vi "yolo-detect-image.vi"() -> ()   [LabVIEW 2017]
uses:
  <vilib>/httpClient/POSTBuffer.vi
  <vilib>/httpClient/LabVIEWHTTPClient.lvlib
panel:
  out "body":string
  out "headers":string
  in  "error in (no error)":errorcluster
  in  "yolo-server \"detect \"endpoint":string="http://localhost:18080/detect"
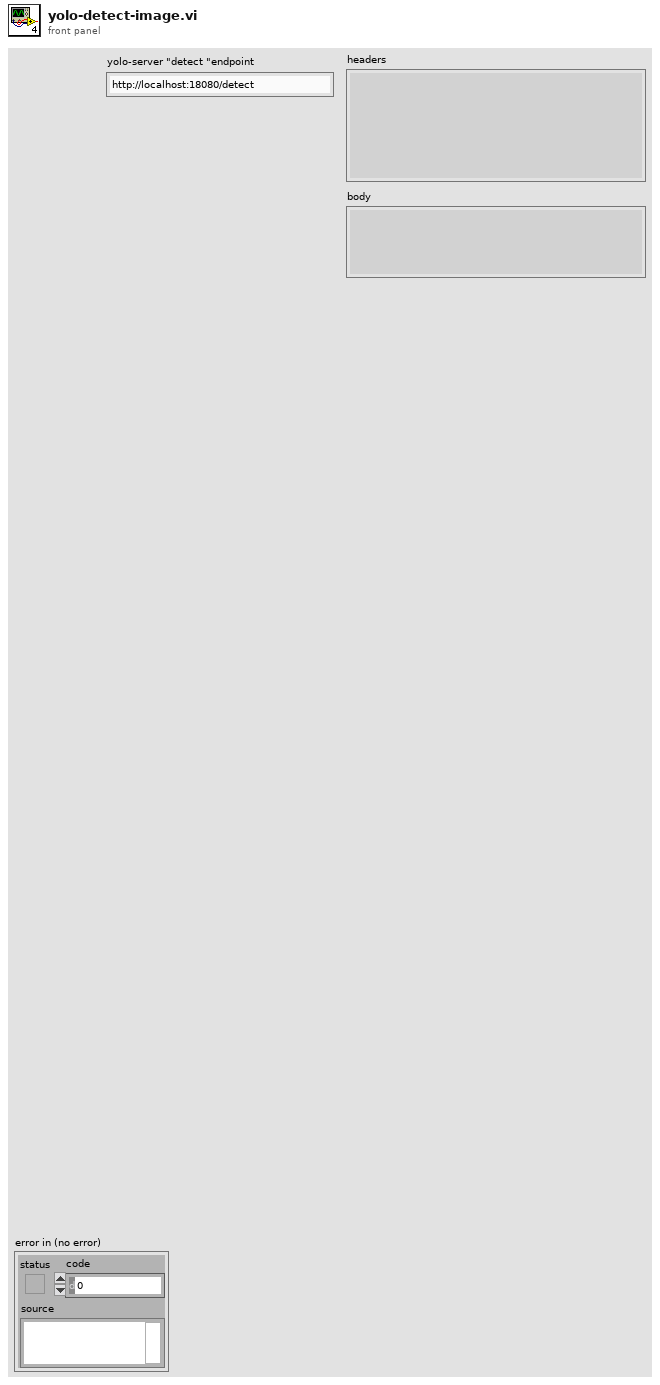
[diagram p1: front panel]
types:
  T1 = typedef "LabVIEWHTTPClient.lvlib/ClientHandle.ctl" = refnum<k1>
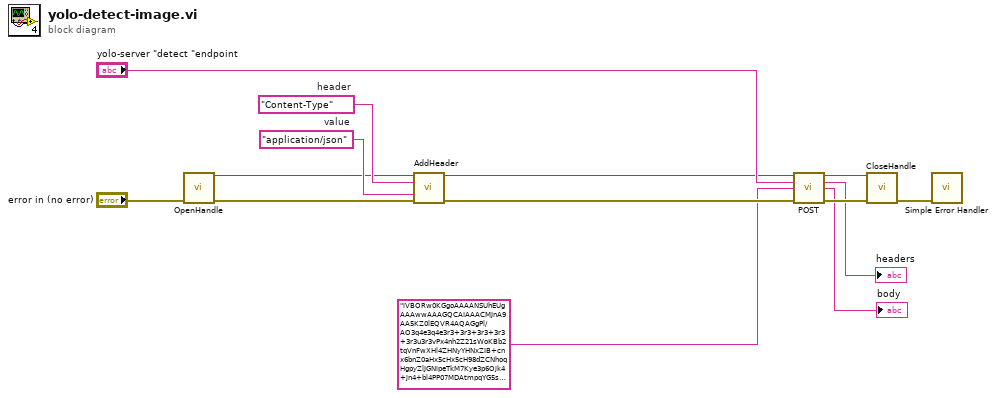
[diagram p0: block diagram]
diagram:
  w14 = "application/json"  # value
  w13 = "Content-Type"  # header
  n1 = call <vilib>:"OpenHandle.vi"("error in (no error)"="error in (no error)") -> ("client handle out"=w7:T1, "error out"=w8:errorcluster)  [unwired: 13 in]
  n2 = call <vilib>:"AddHeader.vi"("client handle"=w7, "header"=w13, "value"=w14, "error in (no error)"=w8) -> ("client handle out"=w4:T1, "error out"=w3:errorcluster)  [unwired: 10 in]
  n3 = call-poly <vilib>:"POST.vi"("client handle"=w4, "url"="yolo-server \"detect \"endpoint", "buffer"="iVBORw0KGgoAAAANSUhEUgAAAwwAAAGQCAIAAACMJnA9AA5KZ0lEQVR4AQAGgPl/AO3q4e3q4e3r3+3r3+3r3+3r3+3r3u3r3vPx4nh2Z21sWoKBb2tqVnFwXHl4ZHNyYHNxZIB+cnx6bnZ0aHx5cHx5cH98dZCNhoqHgpyZlJGNipeTkM7Kye3p6Ojk4+jn4+bl4PP07MDAtmpqYG5sYMLAs+7o3NbQwJ+Wh52VgqqdjKuei7KjjpmKdY5+Z87BrsS+sn16cUJCOikqIh8gGiIlHiMmHxcaERQUDDc1KV5YTJ6VhrWol6WWgbKgirKgiLSeibmkj7ahjq2ciLSjk7msnKeZjId9cauimaqmnXVya2ZnYWBgXmlraIaKiVZVUTAmHDgoGT8vIHNkUcu8p7ChirOli7Oli7SmjLyulL2ul7mqlbytmriomJeHemxeUZCJeYiGd1JTS0BHQEdSTn6JhVtgWSQkGC4mEzMkDUMvFLWhhsCwl4yBa353Z7CtnLGwnrK0n6+woKOnmJuhk5aglZCckoeUi36OhHaGfEZSSF9rX5mhltHZysTKvNTXxOHfyKWfhWtnTJGNcpOPdIF9..." ("string out (base64-encoded)"), "error in (no error)"=w3) -> ("client handle out"=w9:T1, "headers"=→"headers":string, "body"=→"body":string, "error out"=w10:errorcluster)  [unwired: 8 in]
  n4 = call <vilib>:"CloseHandle.vi"("client handle"=w9, "error in (no error)"=w10) -> ("error out"=w2:errorcluster)  [unwired: 13 in]
  n5 = call <vilib>:"Simple Error Handler.vi"("error in (no error)"=w2) -> ()  [unwired: 4 in, 5 out]
